vi "Correction Data 1st.vi"(8 "错误输入":errorcluster, 9 "写入（非为读取）":bool, 10 "Biometry Configuration":T1, 11 "Input Correction Data":dbl[](array[numeric])) -> (0 "错误输出":errorcluster, 3 "Output Correction Data":dbl[](array[numeric]))   [LabVIEW 2015, in "Boimetry Processing.lvlib"]
doc: "读取或者写入轴向扫描距离修正参数（第一部分）。\n读取是：布尔设置为false；\n写入时：布尔设置为true。"
uses:
  Boimetry Processing.lvlib
  Controls/Biometry Configuration.ctl
  <vilib>/Utility/file.llb/Read Delimited Spreadsheet (DBL).vi
  <vilib>/Utility/file.llb/Write Delimited Spreadsheet (DBL).vi
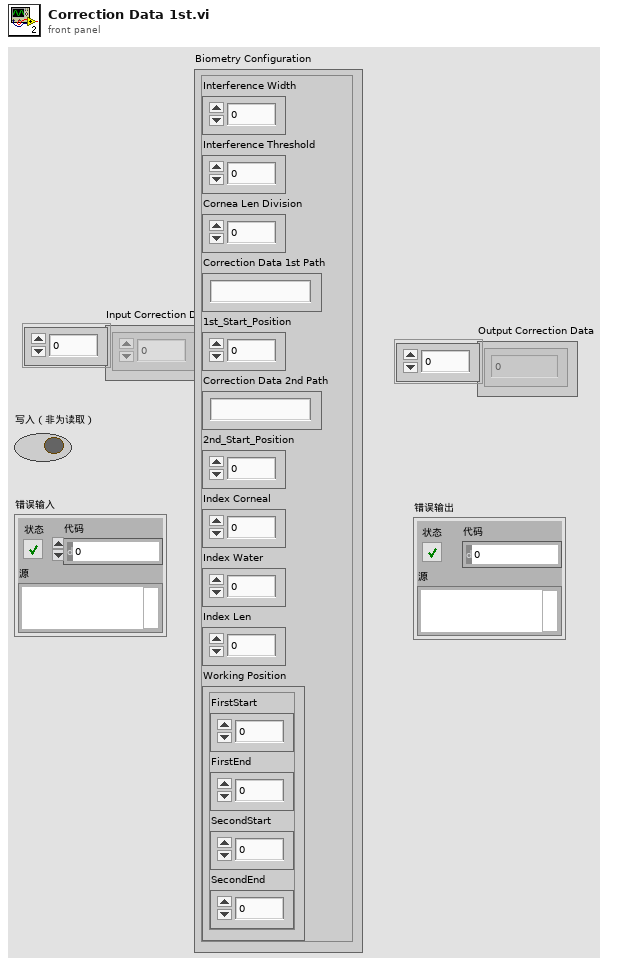
[diagram p1: front panel]
types:
  T1 = typedef "Boimetry Processing.lvlib/Biometry Configuration.ctl" = cluster{"Interference Width":i32, "Interference Threshold":dbl, "Cornea Len Division":i32, "Correction Data 1st Path":string, "1st_Start_Position":dbl, "Correction Data 2nd Path":string, "2nd_Start_Position":dbl, "Index Corneal":dbl, "Index Water":dbl, "Index Len":dbl, "Working Position":cluster{"FirstStart":i32, "FirstEnd":i32, "SecondStart":i32, "SecondEnd":i32}}
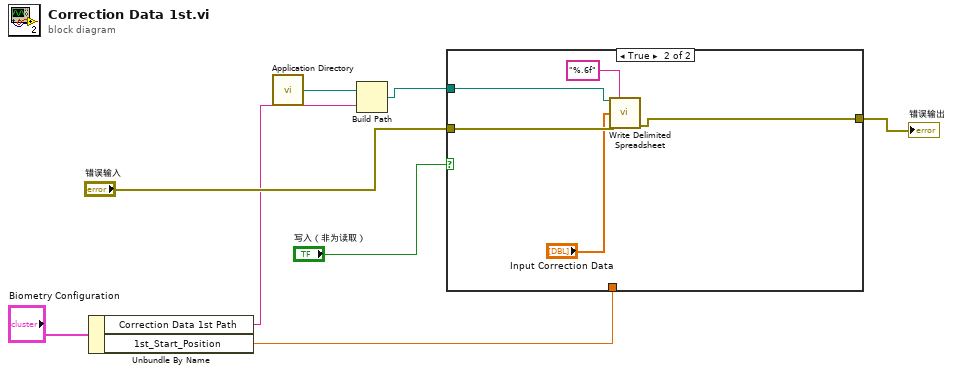
[diagram p0: block diagram]
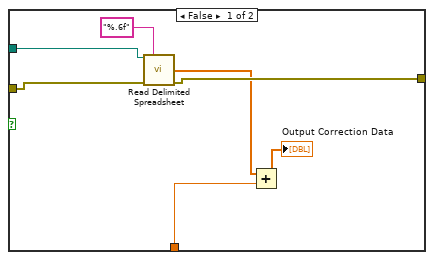
[diagram p2: hidden frame]
diagram:
  n1 = Unbundle By Name("Biometry Configuration") -> ("Correction Data 1st Path"=w2:string, "1st_Start_Position"=w1:dbl)
  n2 = call <vilib>:"Application Directory.vi"() -> ("Application Directory"=w8:path)
  n3 = Build Path(base path=w8, name or relative path=w2) -> (appended path=w6:path)
  n4 = case shown="True" "写入（非为读取）" {
    tunnel: "错误输入" -> [w14 w19]
    tunnel: w6 -> [w15 w20]
    tunnel: [w13 w17] -> w4
    tunnel: w1 -> [w10 _]
    frame False {
      n5 = call-poly <vilib>:"Read Delimited Spreadsheet.vi"("file path (dialog if empty)"=w15, "format (%.3f)"="%.6f", "error in (no error)"=w14) -> ("first row"=w12:dbl[], "error out"=w13:errorcluster)  [unwired: 7 in, 4 out]
      n6 = Add(x=w12, y=w10) -> (x+y=→"Output Correction Data":dbl[])
    }
    frame True {
      n7 = call-poly <vilib>:"Write Delimited Spreadsheet.vi"("file path (dialog if empty)"=w20, "format (%.3f)"="%.6f", "1D data"="Input Correction Data", "error in (no error)"=w19) -> ("error out"=w17:errorcluster)  [unwired: 10 in, 1 out]
    }
  }
  "错误输出" <- w4
